vi "Fetch Waveforms.vi"(8 "error in (no error)":errorcluster, 11 "Fetch Waveforms CFG in":refnum<class "Fetch Waveforms CFG.lvclass">) -> (0 "error out":errorcluster, 2 "Last Waveforms":map{u8, waveform(dbl)}(c390), 3 "Fetch Waveforms CFG out":refnum<class "Fetch Waveforms CFG.lvclass">)   [LabVIEW 2023, in "PXIe-4353.lvlib" / "Fetch Waveforms CFG.lvclass"]
uses:
  Fetch Waveforms CFG.lvclass
  Thermometer/Thermometer DAQmx/Thermometer DAQmx Config/Thermometer DAQmx Config.lvclass/Thermometer DAQmx Config.ctl
  Fetch Waveforms CFG.lvclass/Fetch Waveforms CFG.ctl
  <vilib>/DAQmx/read.llb/DAQmx Read (Analog 1D Wfm NChan NSamp).vi
  <vilib>/DAQmx/miscellaneous.llb/DAQmx Fill In Error Info.vi
  Thermometer/Thermometer DAQmx/Thermometer DAQmx Config/Thermometer DAQmx Config.lvclass
panel:
  out "Waveform Graph":waveform(dbl)[](graph)
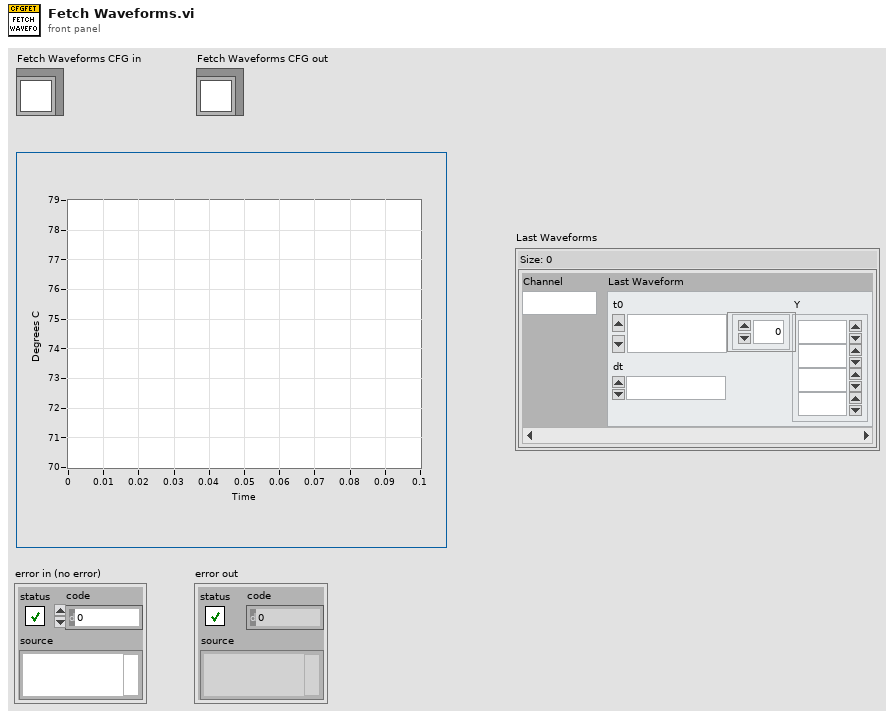
[diagram p1: front panel]
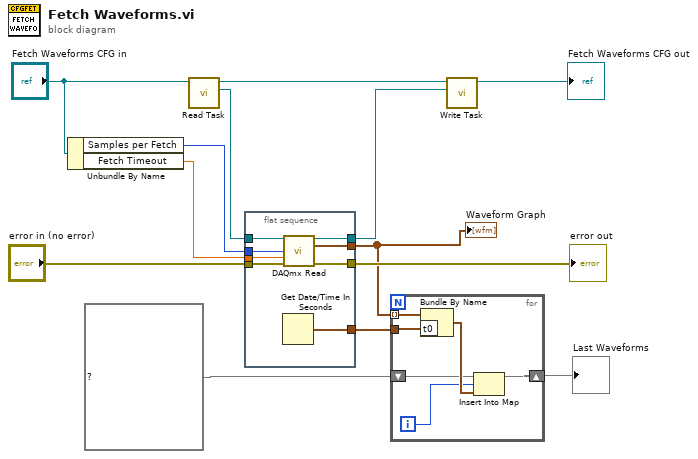
[diagram p0: block diagram]
diagram:
  n1 = Unbundle By Name("Fetch Waveforms CFG in") -> ("Samples per Fetch"=w5:i32, "Fetch Timeout"=w6:dbl)
  n2 = call "Read Task.vi"("Thermometer DAQmx Config in"="Fetch Waveforms CFG in") -> ("Task"=w12:refnum<k21>, "Thermometer DAQmx Config out"=w13:refnum<class "Fetch Waveforms CFG.lvclass">)  [unwired: 8 in, 1 out]
  n3 = flat-sequence {
    tunnel: w12 -> [w21]
    tunnel: "error in (no error)" -> [w20]
    tunnel: [w19] -> w4
    tunnel: [w18] -> w9
    tunnel: [w17] -> w8
    tunnel: w6 -> [w16]
    tunnel: w5 -> [w15]
    tunnel: [w14] -> w3
    frame #0 {
      n4 = Get Date/Time In Seconds() -> (seconds since 1Jan1904=w14:timestamp)
      n5 = call-poly <vilib>:"DAQmx Read.vi"("task/channels in"=w21, "number of samples per channel"=w15, "timeout"=w16, "error in"=w20) -> ("task out"=w18:refnum<k21>, "data"=w19:waveform(dbl)[], "error out"=w17:errorcluster)  [unwired: 9 in]
    }
  }
  n6 = for {
    tunnel: w4 -> [w27] mode=indexing
    tunnel: w3 -> [w26]
    shift-right: [w22] -> w1
    shift-left: map{u8, waveform(dbl)} {} ("Last Waveforms") -> [w23]
    i -> [w24]
    n7 = Bundle By Name(cluster=w27, "t0"=w26) -> (w25:waveform(dbl))
    n8 = Insert Into Map(map in=w23, key=w24, value=w25) -> (map out=w22:map{u8, waveform(dbl)})  [unwired: 2 out]
  }
  "Last Waveforms" <- w1
  n9 = call "Write Task.vi"("Task"=w9, "Thermometer DAQmx Config in"=w13) -> ("Thermometer DAQmx Config out"=→"Fetch Waveforms CFG out":refnum<class "Fetch Waveforms CFG.lvclass">)  [unwired: 8 in, 1 out]
  "error out" <- w8
  "Waveform Graph" <- w4
